vi "CRYExchange Symbol String Sub.vi"(7 "sAction":string, 9 "nData":i32, 10 "sData":string, 11 "Tree in":refnum<vi>) -> (0 "bData Out":bool=TRUE, 1 "nData out":i32=81, 2 "sData out":string, 3 "Tree Out":refnum<vi>)   [LabVIEW 2013]
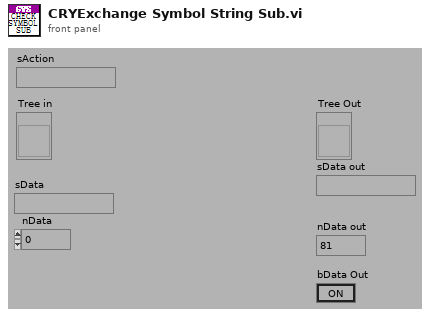
[diagram p1: front panel]
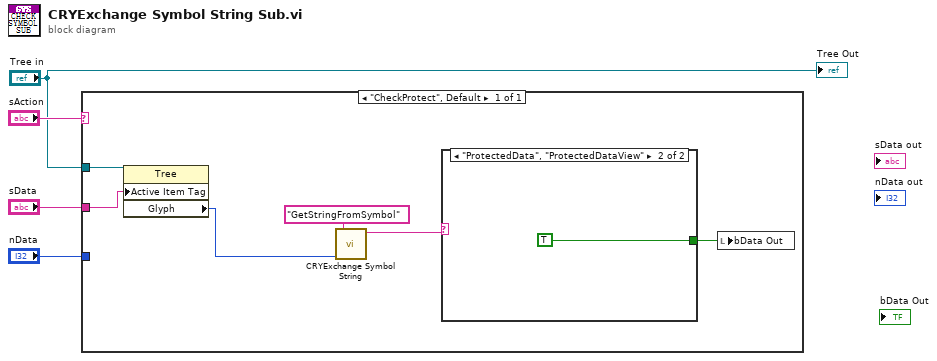
[diagram p0: block diagram]
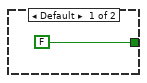
[diagram p2: hidden frame]
diagram:
  n1 = case shown="\"CheckProtect\", Default" "sAction" {
    tunnel: "sData" -> [w6]
    tunnel: "nData" -> [_]
    tunnel: "Tree in" -> [w7]
    frame "CheckProtect", Default {
      n2 = property class="Tree"(reference=w7, "Active Item Tag"=w6) -> ("Glyph"=w5:i32)  [unwired: 1 in, 2 out]
      n3 = call "CRYExchange Symbol String.vi"("nData"=w5, "sAction"="GetStringFromSymbol") -> ("sData out"=w9:string)  [unwired: 8 in, 1 out]
      n4 = case shown="\"ProtectedData\", \"ProtectedDataView\"" w9 {
        tunnel: [FALSE ("bData Out") TRUE ("bData Out")] -> w8
        frame Default {
        }
        frame "ProtectedData", "ProtectedDataView" {
        }
      }
      n5 = local write "bData Out"(w8) -> ()
    }
  }
  "Tree Out" <- "Tree in"
